vi "parse.last_modified.vi"(8 "error in (no error)":errorcluster, 10 "body":string, 11 "comic_class in":refnum<class "comic_class.lvclass">) -> (0 "error out":errorcluster, 3 "comic_class out":refnum<class "comic_class.lvclass">)   [LabVIEW 2024, in "comic_class.lvclass"]
uses:
  comic_class.lvclass
  comic_class.lvclass/comic_class.ctl
  <userlib>/_OpenG.lib/string/string.llb/openg_string.lvlib
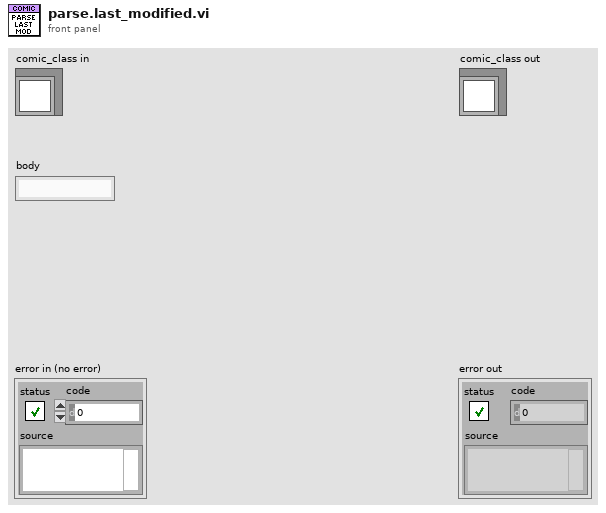
[diagram p1: front panel]
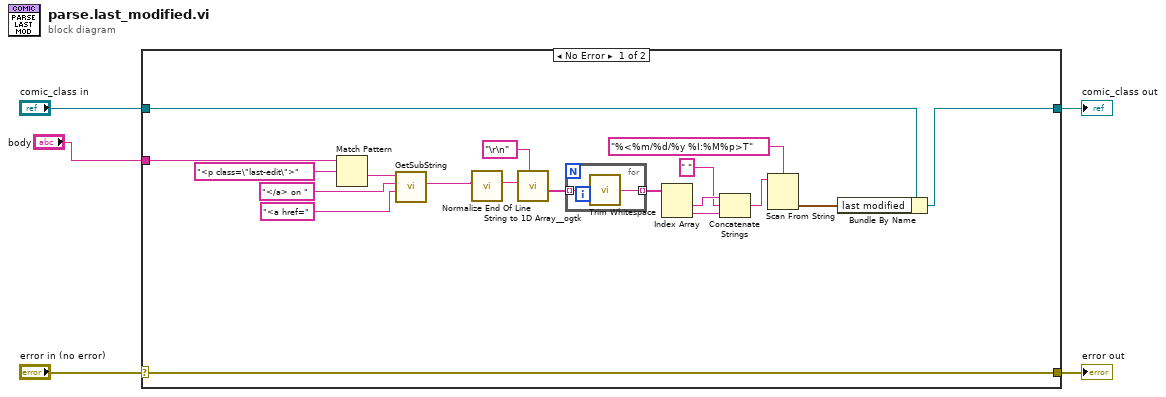
[diagram p0: block diagram]
diagram:
  n1 = case shown="No Error" "error in (no error)" {
    selector: "error in (no error)" -> [w24 w28]
    tunnel: [w24 w28] -> w4
    tunnel: [w7 w27] -> w2
    tunnel: "comic_class in" -> [w8 w27]
    tunnel: "body" -> [w6 _]
    frame No Error {
      n2 = Match Pattern(string=w6, regular expression="<p class=\"last-edit\">") -> (after substring=w22:string)  [unwired: 1 in, 3 out]
      n3 = call "GetSubString.vi"("End Search"="<a href=" ("Start Search"), "Start Search"="</a> on ", "String In"=w22) -> ("Match"=w10:string)  [unwired: 6 in, 2 out]
      n4 = call <vilib>:"Normalize End Of Line.vi"("string in"=w10) -> ("string out"=w17:string)  [unwired: 7 in]
      n5 = call <userlib>:"String to 1D Array__ogtk.vi"("delimiter (Tab)"="\r\n", "string"=w17) -> ("Array of Strings"=w16:string[])  [unwired: 9 in]
      n6 = for {
        tunnel: w16 -> [w26] mode=indexing
        tunnel: [w25] -> w11 mode=indexing
        n7 = call <vilib>:"Trim Whitespace.vi"("string"=w26) -> ("trimmed string"=w25:string)  [unwired: 1 in]
      }
      n8 = Index Array(array=w11) -> (element #1=w15:string, element #2=w14:string)  [unwired: 2 in]
      n9 = Concatenate Strings(w15, " " ("string"), w14) -> (w12:string)
      n10 = Scan From String(format string="%<%m/%d/%y %I:%M%p>T", input string=w12) -> (output 1=w9:timestamp)  [unwired: 3 in, 3 out]
      n11 = Bundle By Name(cluster=w8, "last modified"=w9) -> (w7:refnum<class "comic_class.lvclass">)
    }
    frame Error {
    }
  }
  "error out" <- w4
  "comic_class out" <- w2
